vi "Calibration_And_Constant_Globals.vi"() -> ()   [LabVIEW 2020]
panel:
  in  "Robot_Name":enum16{"Alpha-2022", "Beta-2022"}(ring)
  in  "Copilot_Joystick":string="Copilot_Joystick"
  in  "Pilot_Joystick":string="Pilot_Joystick"
  in  "Robot_Length(in)":dbl=28.0
  in  "Robot_Width(in)":dbl=28.0
  in  "Max_Ground_Speed (ft/s)":dbl=14.0
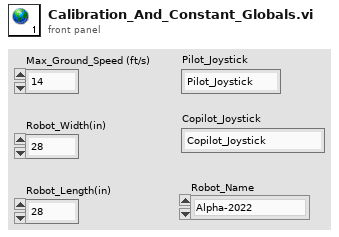
[diagram p1: front panel]
diagram:
